vi "Global 1.vi"() -> ()   [LabVIEW 2010]
panel:
  out "intout":i32
  in  "intin":i32
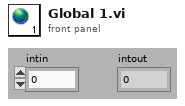
[diagram p1: front panel]
diagram:
